vi "ReportExcel20.vi"(1 "Ürün Parça No":string, 2 "Encoder Testi":bool, 3 "Ürün Seri No":string, 4 "Sıcaklık(°C)":dbl, 9 "Test Sonuçlari":string[][](table)=[["Emk Sabiti", "", "1"], ["R1 (U-V)R", "", "2"], ["R2 (V-W)R", "", "3"], ["R3 (U-W)R", "", "4"], ["L1 (U-V)mH", "", "5"], ["L2 (V-W)mH", "", "6"], ["L3 (U-W)mH", "", "7"]] caption="Test Sonuçları", 11 "error in (no error)":errorcluster, 12 "Sonuc":bool, 14 "Faz Doğrulama Testi":bool) -> (10 "appended path":path, 15 "error out":errorcluster)   [LabVIEW 2021]
uses:
  <vilib>/addons/_office/NI_ReportGenerationToolkit.lvlib
  <vilib>/addons/_office/excel.llb/Excel Easy Table (str).vi
  <vilib>/Utility/NIReport.llb/Excel/NI_Excel.lvclass
  <vilib>/Utility/NIReport.llb/NI_report.lvclass
  <vilib>/Utility/NIReport.llb/Report Type.ctl
  <vilib>/Utility/NIReport.llb/NI_ReportGenerationCore.lvlib
  <vilib>/Utility/NIReport.llb/Append Text Table to Report (wrap).vi
  <vilib>/addons/_office/_exclsub.llb/font.ctl
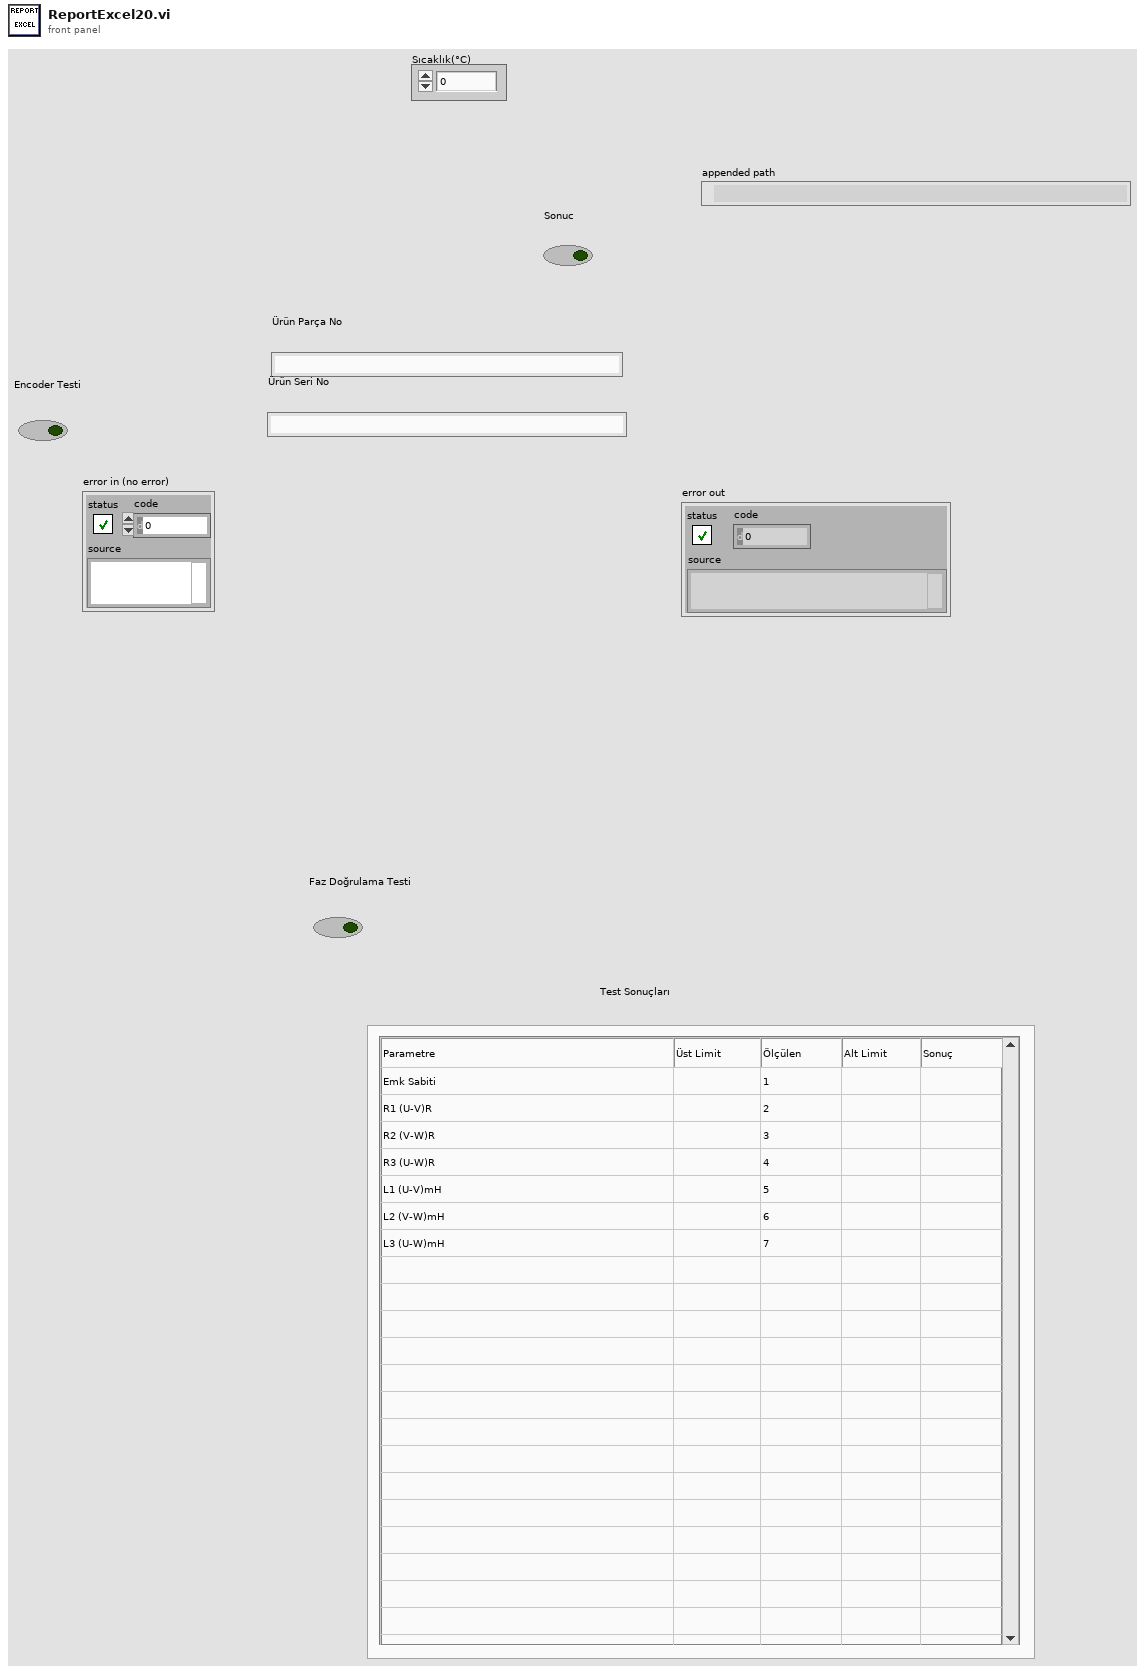
[diagram p1: front panel]
types:
  T1 = typedef "NI_ReportGenerationCore.lvlib/Report Type.ctl" = enum16{"HTML", "Word", "Excel"}
  T2 = enum16{"maximized", "minimized", "normal", "no change"}
  T3 = typedef "NI_ReportGenerationToolkit.lvlib/font.ctl" = cluster{"font name":string, "font size":dbl, "bold":u16, "italic":u16, "underline":u16, "strike through":u16, "font color":u32}
  T4 = cluster{"position (excel)":cluster{"row":i32, "column":i32}, "name (excel)":string, "bookmark (word)":string}
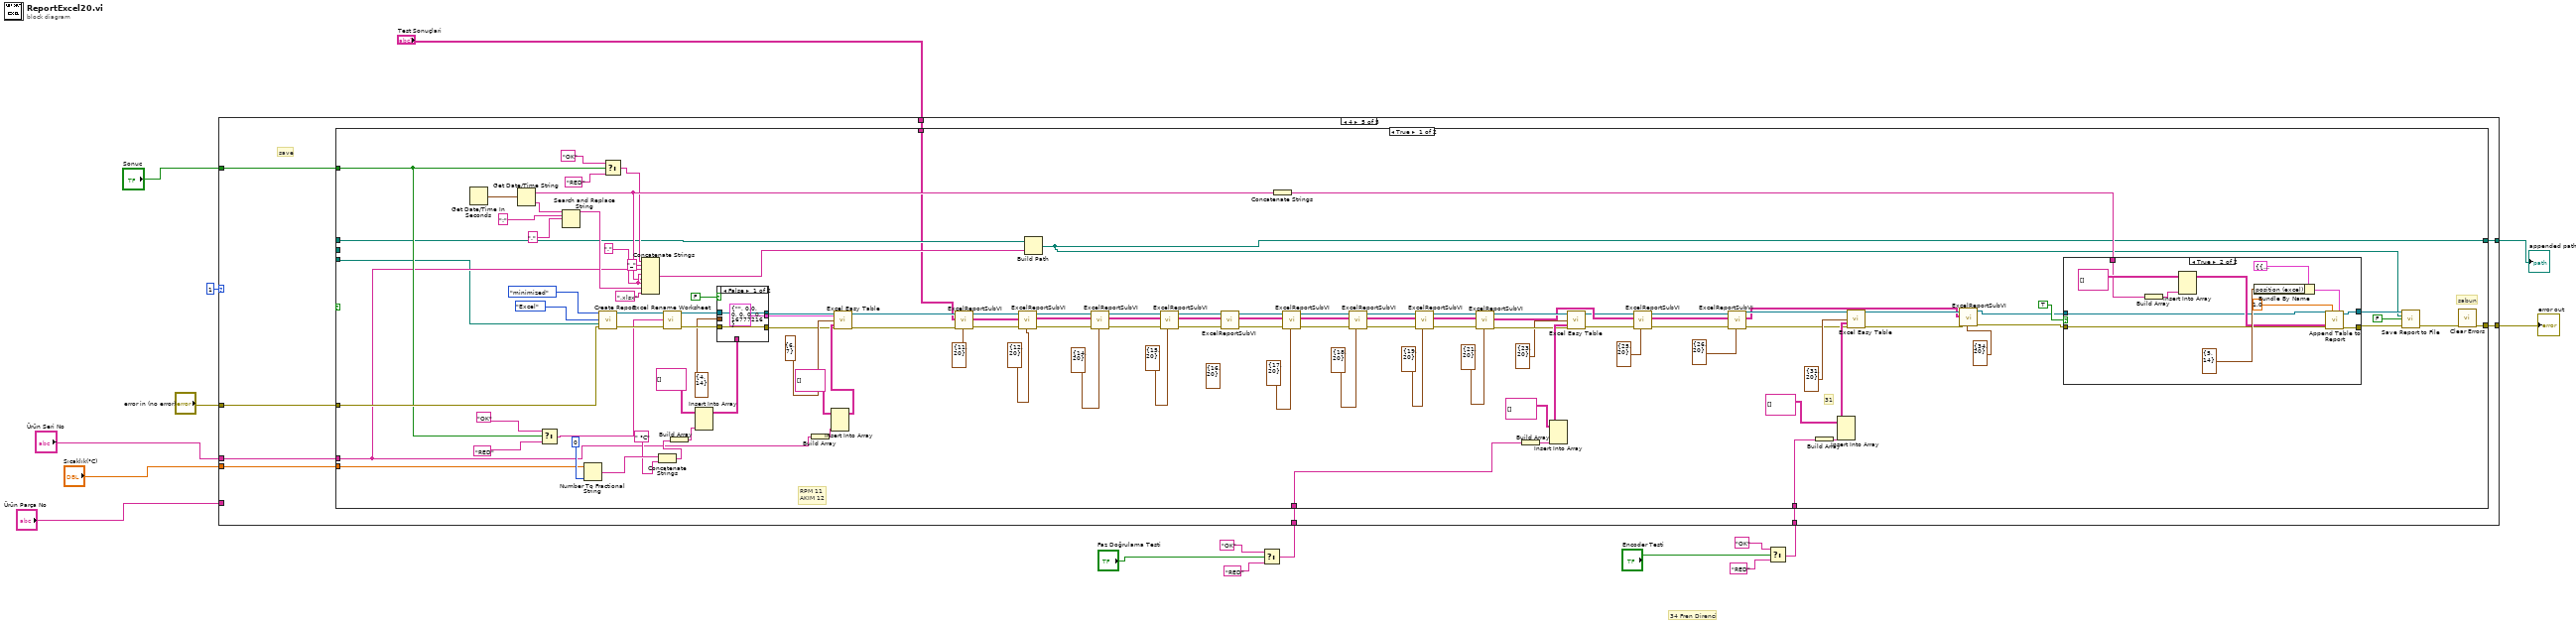
[diagram p0: block diagram]
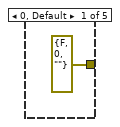
[diagram p2: hidden frame]
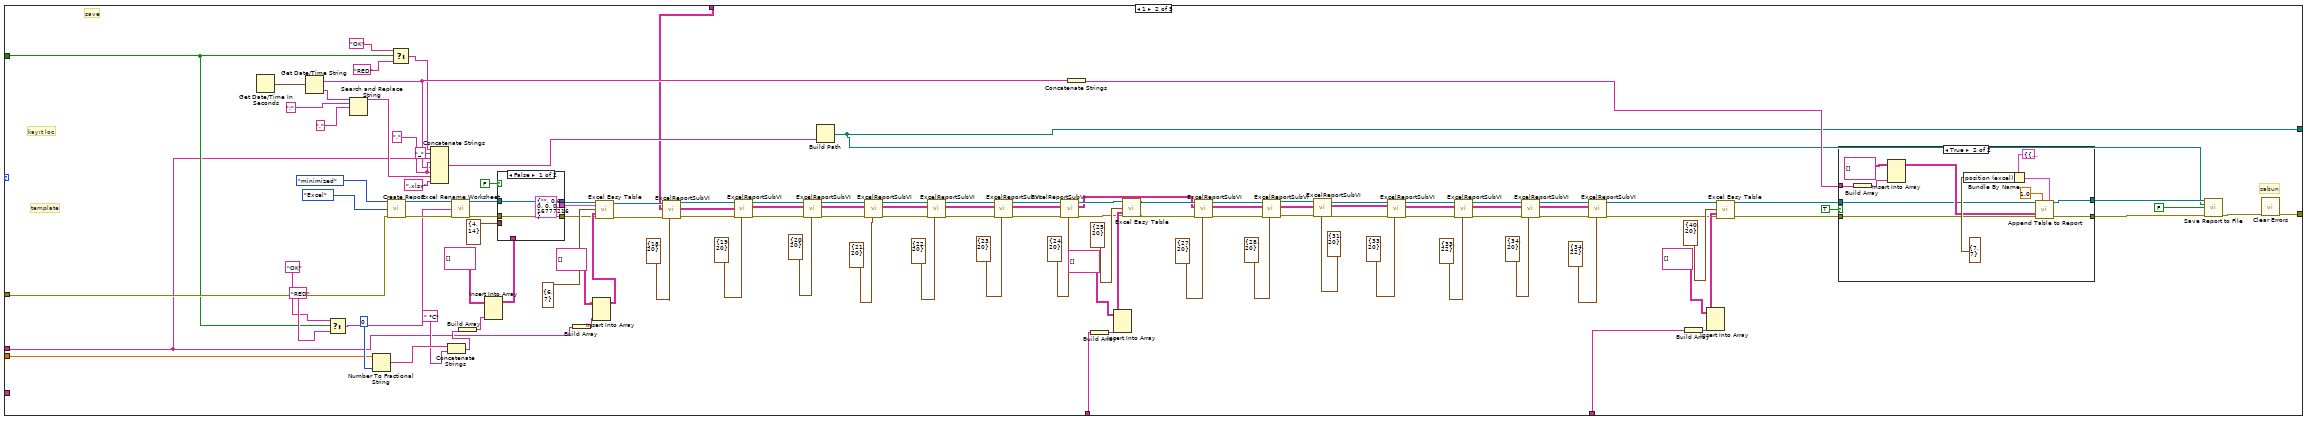
[diagram p3: hidden frame]
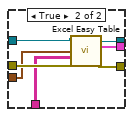
[diagram p4: hidden frame]
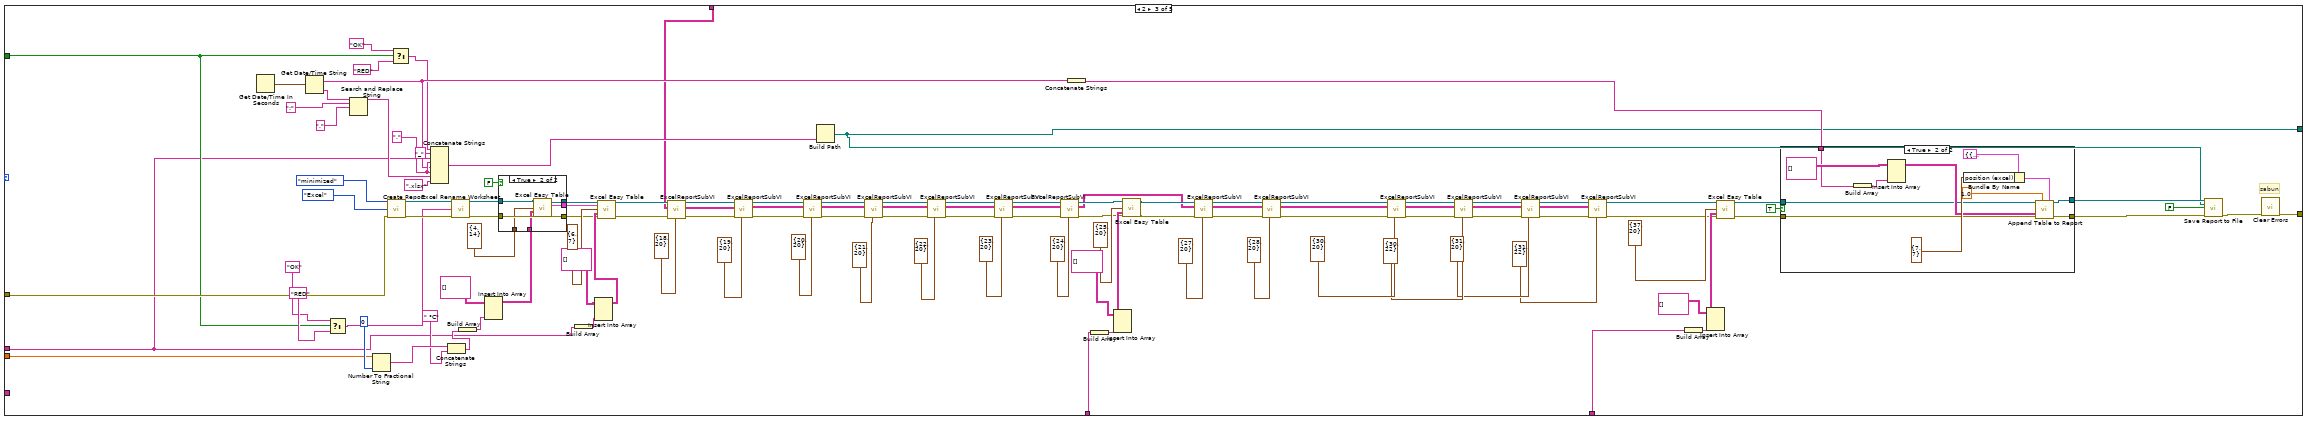
[diagram p6: hidden frame]
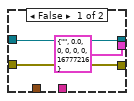
[diagram p7: hidden frame]
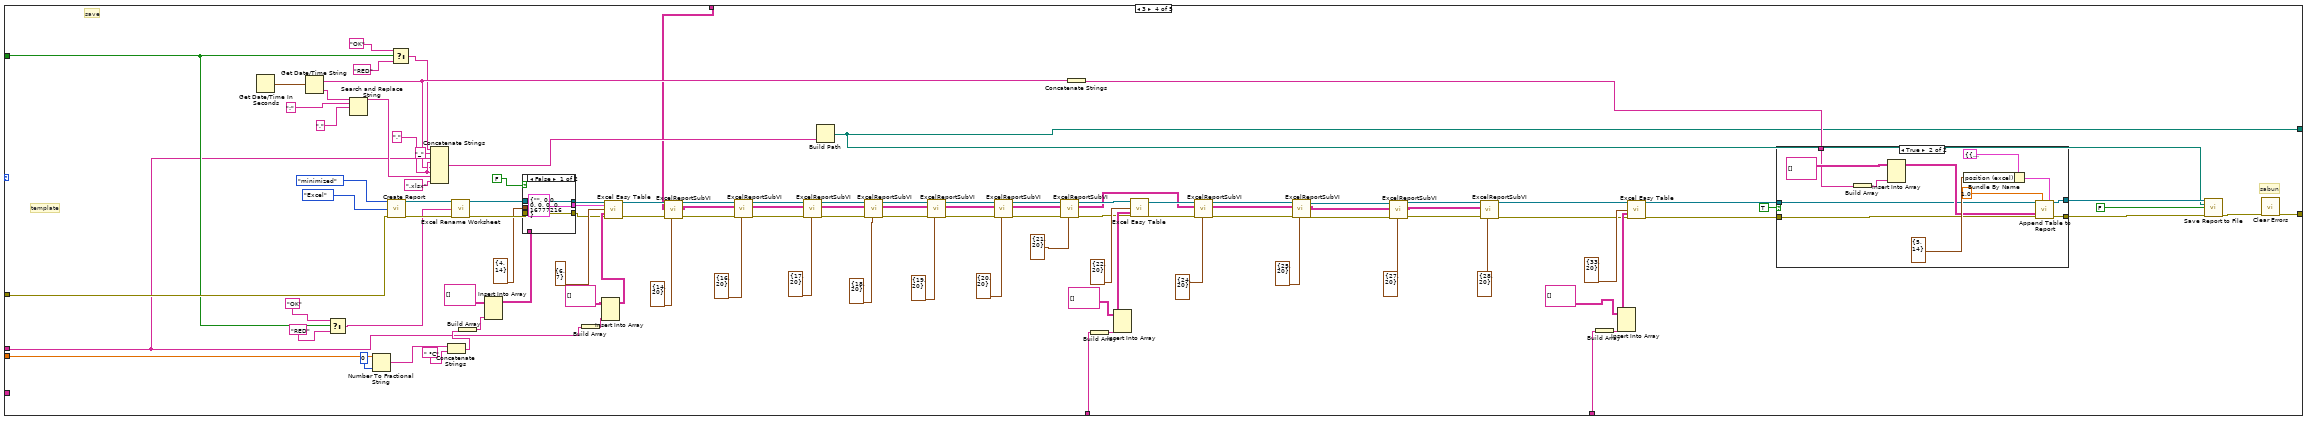
[diagram p9: hidden frame]
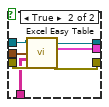
[diagram p10: hidden frame]
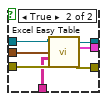
[diagram p12: hidden frame]
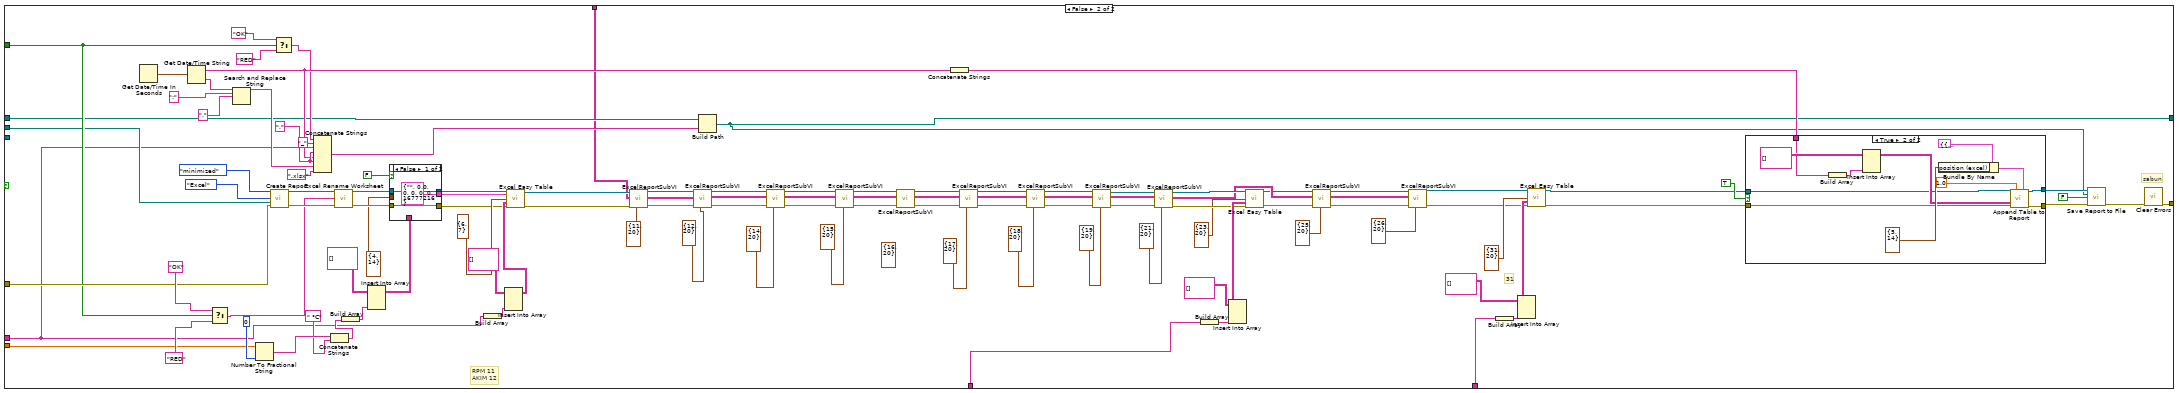
[diagram p14: hidden frame]
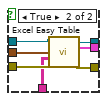
[diagram p15: hidden frame]
diagram:
  # "34 Fren Direnci"
  n1 = Select(t="OK" ("worksheet name (\"\")"), s="Faz Doğrulama Testi", f="RED" ("worksheet name (\"\")")) -> (s? t:f=w13:string)
  n2 = Select(t="OK" ("worksheet name (\"\")"), s="Encoder Testi", f="RED" ("worksheet name (\"\")")) -> (s? t:f=w12:string)
  n3 = case shown="4" 1 {
    tunnel: [errorcluster {"status"=FALSE, "code"=0, "source"=""} ("error out") w108 w252 w398 w466] -> w17
    tunnel: w13 -> [_ w74 w216 w371 w459]
    tunnel: w12 -> [_ w66 w208 w363 w458]
    tunnel: "Sıcaklık(°C)" -> [_ w54 w196 w346 w465]
    tunnel: "error in (no error)" -> [_ w53 w195 w345 w464]
    tunnel: "Sonuc" -> [_ w52 w194 w344 w463]
    tunnel: [_ w51 w193 w343 w462] -> w5
    tunnel: "Ürün Seri No" -> [_ w40 w187 w327 w460]
    tunnel: "Ürün Parça No" -> [_ _ _ _ _]
    tunnel: "Test Sonuçlari" -> [_ w34 w179 w324 w461]
    frame 0, Default {
    }
    frame 1 {
      w132 = "." ("string")
      # "kayıt loc"
      # "save"
      # "template"
      # "sabun"
      n4 = Get Date/Time In Seconds() -> (seconds since 1Jan1904=w139:timestamp)
      n5 = Get Date/Time String(seconds (now)=w139) -> (date string=w129:string, time string=w130:string)  [unwired: 2 in]
      n6 = Select(t="OK" ("worksheet name (\"\")"), s=w52, f="RED" ("worksheet name (\"\")")) -> (s? t:f=w131:string)
      n7 = Search and Replace String(input string=w130, search string=":", replace string="." ("replace string (\"\")")) -> (result string=w125:string)  [unwired: 5 in, 3 out]
      n8 = Number To Fractional String(number=w54, precision (6)=i16 0) -> (F-format string=w115:string)  [unwired: 2 in]
      n9 = call <vilib>:"Create Report.vi"("window state (normal)"=T2."minimized", "report type"=Report_Type."Excel", "error in (no error)"=w53) -> ("report out"=w141:refnum<class "NI_report.lvclass">, "template (empty)"=w49:path, "error out"=w140:errorcluster)  [unwired: 10 in]
      n10 = Select(t="OK" ("worksheet name (\"\")"), s=w52, f="RED" ("worksheet name (\"\")")) -> (s? t:f=w55:string)
      n11 = Concatenate Strings(w55, "_" ("string"), w40, w132, w129, w132, w125, ".xlsx" ("string")) -> (w136:string)
      n12 = Concatenate Strings(w115, " °C" ("string")) -> (w113:string)
      n13 = call <vilib>:"Excel Rename Worksheet.vi"("report in"=w141, "worksheet name (\"\")"=w131, "error in (no error)"=w140) -> ("report out"=w120:refnum<class "NI_report.lvclass">, "error out"=w119:errorcluster)  [unwired: 11 in]
      n14 = Build Array(w113) -> (w116:string[])
      n15 = Insert Into Array(array=string[][] [] ("text data"), new element=w116) -> (w112:string[][])  [unwired: 2 in]
      n16 = case shown="False" FALSE {
        tunnel: w120 -> [w145 w152]
        tunnel: w119 -> [w144 w151]
        tunnel: cluster{"row":i32, "column":i32} {"row"=4, "column"=14} ("start (0, 0)") -> [_ w150]
        tunnel: w112 -> [_ w149]
        tunnel: [w145 w148] -> w43
        tunnel: [w144 w147] -> w42
        tunnel: [T3 {"font name"="", "font size"=0.0, "bold"=0, "italic"=0, "underline"=0, "strike through"=0, "font color"=16777216} ("font out") w146] -> w41
        frame False {
        }
        frame True {
          n17 = call-poly <vilib>:"Excel Easy Table.vi"("report in"=w152, "start (0, 0)"=w150, "text data"=w149, "error in (no error)"=w151) -> ("report out"=w148:refnum<class "NI_report.lvclass">, "font out"=w146:T3, "error out"=w147:errorcluster)  [unwired: 7 in, 2 out]
        }
      }
      n18 = Build Array(w40) -> (w124:string[])
      n19 = Insert Into Array(array=string[][] [] ("text data"), new element=w124) -> (w123:string[][])  [unwired: 2 in]
      n20 = call-poly <vilib>:"Excel Easy Table.vi"("report in"=w43, "font"=w41, "start (0, 0)"=cluster{"row":i32, "column":i32} {"row"=6, "column"=7}, "text data"=w123, "error in (no error)"=w42) -> ("report out"=w38:refnum<class "NI_report.lvclass">, "error out"=w37:errorcluster)  [unwired: 6 in, 3 out]
      n21 = call "ExcelReportSubVI.vi"("start (0, 0)"=cluster{"row":i32, "column":i32} {"row"=18, "column"=20}, "error in (no error)"=w37, "Test İn"=w34, "report in"=w38) -> ("error out"=w35:errorcluster, "Table out"=w33:string[][], "report out"=w36:refnum<class "NI_report.lvclass">)  [unwired: 5 in]
      n22 = call "ExcelReportSubVI.vi"("start (0, 0)"=cluster{"row":i32, "column":i32} {"row"=19, "column"=20}, "error in (no error)"=w35, "Test İn"=w33, "report in"=w36) -> ("error out"=w106:errorcluster, "Table out"=w32:string[][], "report out"=w107:refnum<class "NI_report.lvclass">)  [unwired: 5 in]
      n23 = call "ExcelReportSubVI.vi"("start (0, 0)"=cluster{"row":i32, "column":i32} {"row"=20, "column"=20}, "error in (no error)"=w106, "Test İn"=w32, "report in"=w107) -> ("error out"=w104:errorcluster, "Table out"=w31:string[][], "report out"=w105:refnum<class "NI_report.lvclass">)  [unwired: 5 in]
      n24 = Build Path(name or relative path=w136) -> (base path=w50:path, appended path=w51:path)
      n25 = call "ExcelReportSubVI.vi"("start (0, 0)"=cluster{"row":i32, "column":i32} {"row"=21, "column"=20}, "error in (no error)"=w104, "Test İn"=w31, "report in"=w105) -> ("error out"=w96:errorcluster, "Table out"=w30:string[][], "report out"=w103:refnum<class "NI_report.lvclass">)  [unwired: 5 in]
      n26 = call "ExcelReportSubVI.vi"("start (0, 0)"=cluster{"row":i32, "column":i32} {"row"=22, "column"=20}, "error in (no error)"=w96, "Test İn"=w30, "report in"=w103) -> ("error out"=w95:errorcluster, "Table out"=w29:string[][], "report out"=w102:refnum<class "NI_report.lvclass">)  [unwired: 5 in]
      n27 = call "ExcelReportSubVI.vi"("start (0, 0)"=cluster{"row":i32, "column":i32} {"row"=23, "column"=20}, "error in (no error)"=w95, "Test İn"=w29, "report in"=w102) -> ("error out"=w94:errorcluster, "Table out"=w28:string[][], "report out"=w101:refnum<class "NI_report.lvclass">)  [unwired: 5 in]
      n28 = call "ExcelReportSubVI.vi"("start (0, 0)"=cluster{"row":i32, "column":i32} {"row"=24, "column"=20}, "error in (no error)"=w94, "Test İn"=w28, "report in"=w101) -> ("error out"=w71:errorcluster, "Table out"=w27:string[][], "report out"=w72:refnum<class "NI_report.lvclass">)  [unwired: 5 in]
      n29 = Concatenate Strings(w129) -> (w128:string)
      n30 = Build Array(w74) -> (w75:string[])
      n31 = Insert Into Array(array=string[][] [] ("text data"), new element=w75) -> (w77:string[][])  [unwired: 2 in]
      n32 = call-poly <vilib>:"Excel Easy Table.vi"("report in"=w72, "start (0, 0)"=cluster{"row":i32, "column":i32} {"row"=25, "column"=20}, "text data"=w77, "error in (no error)"=w71) -> ("report out"=w69:refnum<class "NI_report.lvclass">, "error out"=w70:errorcluster)  [unwired: 7 in, 3 out]
      n33 = call "ExcelReportSubVI.vi"("start (0, 0)"=cluster{"row":i32, "column":i32} {"row"=27, "column"=20}, "error in (no error)"=w70, "Test İn"=w27, "report in"=w69) -> ("error out"=w93:errorcluster, "Table out"=w26:string[][], "report out"=w100:refnum<class "NI_report.lvclass">)  [unwired: 5 in]
      n34 = call "ExcelReportSubVI.vi"("start (0, 0)"=cluster{"row":i32, "column":i32} {"row"=28, "column"=20}, "error in (no error)"=w93, "Test İn"=w26, "report in"=w100) -> ("error out"=w47:errorcluster, "Table out"=w25:string[][], "report out"=w48:refnum<class "NI_report.lvclass">)  [unwired: 5 in]
      n35 = call "ExcelReportSubVI.vi"("start (0, 0)"=cluster{"row":i32, "column":i32} {"row"=31, "column"=20}, "error in (no error)"=w47, "Test İn"=w25, "report in"=w48) -> ("error out"=w45:errorcluster, "Table out"=w24:string[][], "report out"=w46:refnum<class "NI_report.lvclass">)  [unwired: 5 in]
      n36 = call "ExcelReportSubVI.vi"("start (0, 0)"=cluster{"row":i32, "column":i32} {"row"=33, "column"=20}, "error in (no error)"=w45, "Test İn"=w24, "report in"=w46) -> ("error out"=w92:errorcluster, "Table out"=w23:string[][], "report out"=w99:refnum<class "NI_report.lvclass">)  [unwired: 5 in]
      n37 = call "ExcelReportSubVI.vi"("start (0, 0)"=cluster{"row":i32, "column":i32} {"row"=33, "column"=22}, "error in (no error)"=w92, "Test İn"=w23, "report in"=w99) -> ("error out"=w91:errorcluster, "Table out"=w22:string[][], "report out"=w98:refnum<class "NI_report.lvclass">)  [unwired: 5 in]
      n38 = call "ExcelReportSubVI.vi"("start (0, 0)"=cluster{"row":i32, "column":i32} {"row"=34, "column"=20}, "error in (no error)"=w91, "Test İn"=w22, "report in"=w98) -> ("error out"=w90:errorcluster, "Table out"=w21:string[][], "report out"=w97:refnum<class "NI_report.lvclass">)  [unwired: 5 in]
      n39 = call "ExcelReportSubVI.vi"("start (0, 0)"=cluster{"row":i32, "column":i32} {"row"=34, "column"=22}, "error in (no error)"=w90, "Test İn"=w21, "report in"=w97) -> ("error out"=w61:errorcluster, "report out"=w62:refnum<class "NI_report.lvclass">)  [unwired: 5 in, 1 out]
      n40 = Build Array(w66) -> (w65:string[])
      n41 = Insert Into Array(array=string[][] [] ("text data"), new element=w65) -> (w63:string[][])  [unwired: 2 in]
      n42 = call-poly <vilib>:"Excel Easy Table.vi"("report in"=w62, "start (0, 0)"=cluster{"row":i32, "column":i32} {"row"=40, "column"=20}, "text data"=w63, "error in (no error)"=w61) -> ("report out"=w60:refnum<class "NI_report.lvclass">, "error out"=w59:errorcluster)  [unwired: 7 in, 3 out]
      n43 = case shown="True" TRUE {
        tunnel: w128 -> [_ w164]
        tunnel: [w154 w158] -> w127
        tunnel: [w153 w157] -> w126
        tunnel: w60 -> [w154 w156]
        tunnel: w59 -> [w153 w155]
        frame False {
        }
        frame True {
          n44 = Build Array(w164) -> (w165:string[])
          n45 = Insert Into Array(array=string[][] [] ("text data"), new element=w165) -> (w159:string[][])  [unwired: 2 in]
          n46 = Bundle By Name(cluster=T4 {"position (excel)"={"row"=0, "column"=0}, "name (excel)"="", "bookmark (word)"=""} ("MS Office parameters"), "position (excel)"=cluster{"row":i32, "column":i32} {"row"=7, "column"=7} ("start (0, 0)")) -> (w161:T4)
          n47 = call-poly <vilib>:"Append Table to Report.vi"("report in"=w156, "column width (1)"=1.0, "MS Office parameters"=w161, "text data"=w159, "error in (no error)"=w155) -> ("report out"=w158:refnum<class "NI_report.lvclass">, "error out"=w157:errorcluster)  [unwired: 7 in, 2 out]
        }
      }
      n48 = call-dynamic "Save Report to File.vi"("report in"=w127, "report file path"=w51, "prompt to replace? (F)"=FALSE, "error in (no error)"=w126) -> ("error out"=w109:errorcluster)  [unwired: 10 in, 1 out]
      n49 = call <vilib>:"Clear Errors.vi"("error in (no error)"=w109) -> ("error out"=w108:errorcluster)  [unwired: 5 in, 1 out]
    }
    frame 2 {
      w276 = "." ("string")
      # "sabun"
      n50 = Get Date/Time In Seconds() -> (seconds since 1Jan1904=w283:timestamp)
      n51 = Get Date/Time String(seconds (now)=w283) -> (date string=w273:string, time string=w274:string)  [unwired: 2 in]
      n52 = Select(t="OK" ("worksheet name (\"\")"), s=w194, f="RED" ("worksheet name (\"\")")) -> (s? t:f=w275:string)
      n53 = Search and Replace String(input string=w274, search string=":", replace string="." ("replace string (\"\")")) -> (result string=w269:string)  [unwired: 5 in, 3 out]
      n54 = Number To Fractional String(number=w196, precision (6)=i16 0) -> (F-format string=w259:string)  [unwired: 2 in]
      n55 = call <vilib>:"Create Report.vi"("window state (normal)"=T2."minimized", "report type"=Report_Type."Excel", "error in (no error)"=w195) -> ("report out"=w285:refnum<class "NI_report.lvclass">, "template (empty)"=w191:path, "error out"=w284:errorcluster)  [unwired: 10 in]
      n56 = Select(t="OK" ("worksheet name (\"\")"), s=w194, f="RED" ("worksheet name (\"\")")) -> (s? t:f=w197:string)
      n57 = Concatenate Strings(w197, "_" ("string"), w187, w276, w273, w276, w269, ".xlsx" ("string")) -> (w280:string)
      n58 = Concatenate Strings(w259, " °C" ("string")) -> (w257:string)
      n59 = call <vilib>:"Excel Rename Worksheet.vi"("report in"=w285, "worksheet name (\"\")"=w275, "error in (no error)"=w284) -> ("report out"=w264:refnum<class "NI_report.lvclass">, "error out"=w263:errorcluster)  [unwired: 11 in]
      n60 = Build Array(w257) -> (w260:string[])
      n61 = Insert Into Array(array=string[][] [] ("text data"), new element=w260) -> (w256:string[][])  [unwired: 2 in]
      n62 = case shown="True" FALSE {
        tunnel: w264 -> [w289 w296]
        tunnel: w263 -> [w288 w295]
        tunnel: cluster{"row":i32, "column":i32} {"row"=4, "column"=14} ("start (0, 0)") -> [_ w294]
        tunnel: w256 -> [_ w293]
        tunnel: [w289 w292] -> w190
        tunnel: [w288 w291] -> w189
        tunnel: [T3 {"font name"="", "font size"=0.0, "bold"=0, "italic"=0, "underline"=0, "strike through"=0, "font color"=16777216} ("font out") w290] -> w188
        frame False {
        }
        frame True {
          n63 = call-poly <vilib>:"Excel Easy Table.vi"("report in"=w296, "start (0, 0)"=w294, "text data"=w293, "error in (no error)"=w295) -> ("report out"=w292:refnum<class "NI_report.lvclass">, "font out"=w290:T3, "error out"=w291:errorcluster)  [unwired: 7 in, 2 out]
        }
      }
      n64 = Build Array(w187) -> (w268:string[])
      n65 = Insert Into Array(array=string[][] [] ("text data"), new element=w268) -> (w267:string[][])  [unwired: 2 in]
      n66 = call-poly <vilib>:"Excel Easy Table.vi"("report in"=w190, "font"=w188, "start (0, 0)"=cluster{"row":i32, "column":i32} {"row"=6, "column"=7}, "text data"=w267, "error in (no error)"=w189) -> ("report out"=w185:refnum<class "NI_report.lvclass">, "error out"=w183:errorcluster)  [unwired: 6 in, 3 out]
      n67 = call "ExcelReportSubVI.vi"("start (0, 0)"=cluster{"row":i32, "column":i32} {"row"=18, "column"=20}, "error in (no error)"=w183, "Test İn"=w179, "report in"=w185) -> ("error out"=w182:errorcluster, "Table out"=w180:string[][], "report out"=w184:refnum<class "NI_report.lvclass">)  [unwired: 5 in]
      n68 = call "ExcelReportSubVI.vi"("start (0, 0)"=cluster{"row":i32, "column":i32} {"row"=19, "column"=20}, "error in (no error)"=w182, "Test İn"=w180, "report in"=w184) -> ("error out"=w250:errorcluster, "Table out"=w178:string[][], "report out"=w251:refnum<class "NI_report.lvclass">)  [unwired: 5 in]
      n69 = call "ExcelReportSubVI.vi"("start (0, 0)"=cluster{"row":i32, "column":i32} {"row"=20, "column"=20}, "error in (no error)"=w250, "Test İn"=w178, "report in"=w251) -> ("error out"=w248:errorcluster, "Table out"=w177:string[][], "report out"=w249:refnum<class "NI_report.lvclass">)  [unwired: 5 in]
      n70 = Build Path(name or relative path=w280) -> (base path=w192:path, appended path=w193:path)
      n71 = call "ExcelReportSubVI.vi"("start (0, 0)"=cluster{"row":i32, "column":i32} {"row"=21, "column"=20}, "error in (no error)"=w248, "Test İn"=w177, "report in"=w249) -> ("error out"=w239:errorcluster, "Table out"=w176:string[][], "report out"=w247:refnum<class "NI_report.lvclass">)  [unwired: 5 in]
      n72 = call "ExcelReportSubVI.vi"("start (0, 0)"=cluster{"row":i32, "column":i32} {"row"=22, "column"=20}, "error in (no error)"=w239, "Test İn"=w176, "report in"=w247) -> ("error out"=w238:errorcluster, "Table out"=w175:string[][], "report out"=w246:refnum<class "NI_report.lvclass">)  [unwired: 5 in]
      n73 = call "ExcelReportSubVI.vi"("start (0, 0)"=cluster{"row":i32, "column":i32} {"row"=23, "column"=20}, "error in (no error)"=w238, "Test İn"=w175, "report in"=w246) -> ("error out"=w237:errorcluster, "Table out"=w174:string[][], "report out"=w245:refnum<class "NI_report.lvclass">)  [unwired: 5 in]
      n74 = call "ExcelReportSubVI.vi"("start (0, 0)"=cluster{"row":i32, "column":i32} {"row"=24, "column"=20}, "error in (no error)"=w237, "Test İn"=w174, "report in"=w245) -> ("error out"=w213:errorcluster, "Table out"=w173:string[][], "report out"=w214:refnum<class "NI_report.lvclass">)  [unwired: 5 in]
      n75 = Concatenate Strings(w273) -> (w272:string)
      n76 = Build Array(w216) -> (w217:string[])
      n77 = Insert Into Array(array=string[][] [] ("text data"), new element=w217) -> (w219:string[][])  [unwired: 2 in]
      n78 = call-poly <vilib>:"Excel Easy Table.vi"("report in"=w214, "start (0, 0)"=cluster{"row":i32, "column":i32} {"row"=25, "column"=20}, "text data"=w219, "error in (no error)"=w213) -> ("report out"=w211:refnum<class "NI_report.lvclass">, "error out"=w212:errorcluster)  [unwired: 7 in, 3 out]
      n79 = call "ExcelReportSubVI.vi"("start (0, 0)"=cluster{"row":i32, "column":i32} {"row"=27, "column"=20}, "error in (no error)"=w212, "Test İn"=w173, "report in"=w211) -> ("error out"=w236:errorcluster, "Table out"=w172:string[][], "report out"=w244:refnum<class "NI_report.lvclass">)  [unwired: 5 in]
      n80 = call "ExcelReportSubVI.vi"("start (0, 0)"=cluster{"row":i32, "column":i32} {"row"=28, "column"=20}, "error in (no error)"=w236, "Test İn"=w172, "report in"=w244) -> ("error out"=w235:errorcluster, "Table out"=w171:string[][], "report out"=w243:refnum<class "NI_report.lvclass">)  [unwired: 5 in]
      n81 = call "ExcelReportSubVI.vi"("start (0, 0)"=cluster{"row":i32, "column":i32} {"row"=30, "column"=20}, "error in (no error)"=w235, "Test İn"=w171, "report in"=w243) -> ("error out"=w234:errorcluster, "Table out"=w170:string[][], "report out"=w242:refnum<class "NI_report.lvclass">)  [unwired: 5 in]
      n82 = call "ExcelReportSubVI.vi"("start (0, 0)"=cluster{"row":i32, "column":i32} {"row"=30, "column"=22}, "error in (no error)"=w234, "Test İn"=w170, "report in"=w242) -> ("error out"=w233:errorcluster, "Table out"=w169:string[][], "report out"=w241:refnum<class "NI_report.lvclass">)  [unwired: 5 in]
      n83 = call "ExcelReportSubVI.vi"("start (0, 0)"=cluster{"row":i32, "column":i32} {"row"=31, "column"=20}, "error in (no error)"=w233, "Test İn"=w169, "report in"=w241) -> ("error out"=w232:errorcluster, "Table out"=w168:string[][], "report out"=w240:refnum<class "NI_report.lvclass">)  [unwired: 5 in]
      n84 = call "ExcelReportSubVI.vi"("start (0, 0)"=cluster{"row":i32, "column":i32} {"row"=31, "column"=22}, "error in (no error)"=w232, "Test İn"=w168, "report in"=w240) -> ("error out"=w203:errorcluster, "report out"=w204:refnum<class "NI_report.lvclass">)  [unwired: 5 in, 1 out]
      n85 = Build Array(w208) -> (w207:string[])
      n86 = Insert Into Array(array=string[][] [] ("text data"), new element=w207) -> (w205:string[][])  [unwired: 2 in]
      n87 = call-poly <vilib>:"Excel Easy Table.vi"("report in"=w204, "start (0, 0)"=cluster{"row":i32, "column":i32} {"row"=37, "column"=20}, "text data"=w205, "error in (no error)"=w203) -> ("report out"=w202:refnum<class "NI_report.lvclass">, "error out"=w201:errorcluster)  [unwired: 7 in, 3 out]
      n88 = case shown="True" TRUE {
        tunnel: w272 -> [_ w308]
        tunnel: [w298 w302] -> w271
        tunnel: [w297 w301] -> w270
        tunnel: w202 -> [w298 w300]
        tunnel: w201 -> [w297 w299]
        frame False {
        }
        frame True {
          n89 = Build Array(w308) -> (w309:string[])
          n90 = Insert Into Array(array=string[][] [] ("text data"), new element=w309) -> (w303:string[][])  [unwired: 2 in]
          n91 = Bundle By Name(cluster=T4 {"position (excel)"={"row"=0, "column"=0}, "name (excel)"="", "bookmark (word)"=""} ("MS Office parameters"), "position (excel)"=cluster{"row":i32, "column":i32} {"row"=7, "column"=7} ("start (0, 0)")) -> (w305:T4)
          n92 = call-poly <vilib>:"Append Table to Report.vi"("report in"=w300, "column width (1)"=1.0, "MS Office parameters"=w305, "text data"=w303, "error in (no error)"=w299) -> ("report out"=w302:refnum<class "NI_report.lvclass">, "error out"=w301:errorcluster)  [unwired: 7 in, 2 out]
        }
      }
      n93 = call-dynamic "Save Report to File.vi"("report in"=w271, "report file path"=w193, "prompt to replace? (F)"=FALSE, "error in (no error)"=w270) -> ("error out"=w253:errorcluster)  [unwired: 10 in, 1 out]
      n94 = call <vilib>:"Clear Errors.vi"("error in (no error)"=w253) -> ("error out"=w252:errorcluster)  [unwired: 5 in, 1 out]
    }
    frame 3 {
      w421 = "." ("string")
      # "save"
      # "template"
      # "sabun"
      n95 = Get Date/Time In Seconds() -> (seconds since 1Jan1904=w428:timestamp)
      n96 = Get Date/Time String(seconds (now)=w428) -> (date string=w419:string, time string=w311:string)  [unwired: 2 in]
      n97 = Select(t="OK" ("worksheet name (\"\")"), s=w344, f="RED" ("worksheet name (\"\")")) -> (s? t:f=w420:string)
      n98 = Search and Replace String(input string=w311, search string=":", replace string="." ("replace string (\"\")")) -> (result string=w415:string)  [unwired: 5 in, 3 out]
      n99 = Number To Fractional String(number=w346, precision (6)=i16 0) -> (F-format string=w405:string)  [unwired: 2 in]
      n100 = call <vilib>:"Create Report.vi"("window state (normal)"=T2."minimized", "report type"=Report_Type."Excel", "error in (no error)"=w345) -> ("report out"=w430:refnum<class "NI_report.lvclass">, "template (empty)"=w341:path, "error out"=w429:errorcluster)  [unwired: 10 in]
      n101 = Select(t="OK" ("worksheet name (\"\")"), s=w344, f="RED" ("worksheet name (\"\")")) -> (s? t:f=w354:string)
      n102 = Concatenate Strings(w354, "_" ("string"), w327, w421, w419, w421, w415, ".xlsx" ("string")) -> (w425:string)
      n103 = Concatenate Strings(w405, " °C" ("string")) -> (w403:string)
      n104 = call <vilib>:"Excel Rename Worksheet.vi"("report in"=w430, "worksheet name (\"\")"=w420, "error in (no error)"=w429) -> ("report out"=w410:refnum<class "NI_report.lvclass">, "error out"=w409:errorcluster)  [unwired: 11 in]
      n105 = Build Array(w403) -> (w406:string[])
      n106 = Insert Into Array(array=string[][] [] ("text data"), new element=w406) -> (w402:string[][])  [unwired: 2 in]
      n107 = case shown="False" FALSE {
        tunnel: w410 -> [w434 w441]
        tunnel: w409 -> [w433 w440]
        tunnel: cluster{"row":i32, "column":i32} {"row"=4, "column"=14} ("start (0, 0)") -> [_ w439]
        tunnel: w402 -> [_ w438]
        tunnel: [w434 w437] -> w330
        tunnel: [w433 w436] -> w329
        tunnel: [T3 {"font name"="", "font size"=0.0, "bold"=0, "italic"=0, "underline"=0, "strike through"=0, "font color"=16777216} ("font out") w435] -> w328
        frame False {
        }
        frame True {
          n108 = call-poly <vilib>:"Excel Easy Table.vi"("report in"=w441, "start (0, 0)"=w439, "text data"=w438, "error in (no error)"=w440) -> ("report out"=w437:refnum<class "NI_report.lvclass">, "font out"=w435:T3, "error out"=w436:errorcluster)  [unwired: 7 in, 2 out]
        }
      }
      n109 = Build Array(w327) -> (w414:string[])
      n110 = Insert Into Array(array=string[][] [] ("text data"), new element=w414) -> (w413:string[][])  [unwired: 2 in]
      n111 = call-poly <vilib>:"Excel Easy Table.vi"("report in"=w330, "font"=w328, "start (0, 0)"=cluster{"row":i32, "column":i32} {"row"=6, "column"=7}, "text data"=w413, "error in (no error)"=w329) -> ("report out"=w397:refnum<class "NI_report.lvclass">, "error out"=w396:errorcluster)  [unwired: 6 in, 3 out]
      n112 = call "ExcelReportSubVI.vi"("start (0, 0)"=cluster{"row":i32, "column":i32} {"row"=14, "column"=20}, "Test İn"=w324) -> ("Table out"=w323:string[][], "Yazılacak Parametre"=w325:string)  [unwired: 6 in, 2 out]
      n113 = call "ExcelReportSubVI.vi"("start (0, 0)"=cluster{"row":i32, "column":i32} {"row"=16, "column"=20}, "error in (no error)"=w396, "Test İn"=w323, "report in"=w397) -> ("error out"=w394:errorcluster, "Table out"=w322:string[][], "report out"=w395:refnum<class "NI_report.lvclass">, "Yazılacak Parametre"=w353:string)  [unwired: 4 in]
      n114 = call "ExcelReportSubVI.vi"("start (0, 0)"=cluster{"row":i32, "column":i32} {"row"=17, "column"=20}, "error in (no error)"=w394, "Test İn"=w322, "report in"=w395) -> ("error out"=w392:errorcluster, "Table out"=w321:string[][], "report out"=w393:refnum<class "NI_report.lvclass">, "Yazılacak Parametre"=w352:string)  [unwired: 4 in]
      n115 = Build Path(name or relative path=w425) -> (base path=w342:path, appended path=w343:path)
      n116 = call "ExcelReportSubVI.vi"("start (0, 0)"=cluster{"row":i32, "column":i32} {"row"=18, "column"=20}, "error in (no error)"=w392, "Test İn"=w321, "report in"=w393) -> ("error out"=w387:errorcluster, "Table out"=w320:string[][], "report out"=w391:refnum<class "NI_report.lvclass">, "Yazılacak Parametre"=w351:string)  [unwired: 4 in]
      n117 = call "ExcelReportSubVI.vi"("start (0, 0)"=cluster{"row":i32, "column":i32} {"row"=19, "column"=20}, "error in (no error)"=w387, "Test İn"=w320, "report in"=w391) -> ("error out"=w386:errorcluster, "Table out"=w319:string[][], "report out"=w390:refnum<class "NI_report.lvclass">, "Yazılacak Parametre"=w350:string)  [unwired: 4 in]
      n118 = call "ExcelReportSubVI.vi"("start (0, 0)"=cluster{"row":i32, "column":i32} {"row"=20, "column"=20}, "error in (no error)"=w386, "Test İn"=w319, "report in"=w390) -> ("error out"=w385:errorcluster, "Table out"=w318:string[][], "report out"=w389:refnum<class "NI_report.lvclass">, "Yazılacak Parametre"=w349:string)  [unwired: 4 in]
      n119 = call "ExcelReportSubVI.vi"("start (0, 0)"=cluster{"row":i32, "column":i32} {"row"=21, "column"=20}, "error in (no error)"=w385, "Test İn"=w318, "report in"=w389) -> ("error out"=w368:errorcluster, "Table out"=w317:string[][], "report out"=w369:refnum<class "NI_report.lvclass">, "Yazılacak Parametre"=w348:string)  [unwired: 4 in]
      n120 = Concatenate Strings(w419) -> (w418:string)
      n121 = Build Array(w371) -> (w372:string[])
      n122 = Insert Into Array(array=string[][] [] ("text data"), new element=w372) -> (w374:string[][])  [unwired: 2 in]
      n123 = call-poly <vilib>:"Excel Easy Table.vi"("report in"=w369, "start (0, 0)"=cluster{"row":i32, "column":i32} {"row"=22, "column"=20}, "text data"=w374, "error in (no error)"=w368) -> ("report out"=w366:refnum<class "NI_report.lvclass">, "error out"=w367:errorcluster)  [unwired: 7 in, 3 out]
      n124 = call "ExcelReportSubVI.vi"("start (0, 0)"=cluster{"row":i32, "column":i32} {"row"=24, "column"=20}, "error in (no error)"=w367, "Test İn"=w317, "report in"=w366) -> ("error out"=w384:errorcluster, "Table out"=w316:string[][], "report out"=w388:refnum<class "NI_report.lvclass">, "Yazılacak Parametre"=w375:string)  [unwired: 4 in]
      n125 = call "ExcelReportSubVI.vi"("start (0, 0)"=cluster{"row":i32, "column":i32} {"row"=25, "column"=20}, "error in (no error)"=w384, "Test İn"=w316, "report in"=w388) -> ("error out"=w337:errorcluster, "Table out"=w315:string[][], "report out"=w338:refnum<class "NI_report.lvclass">, "Yazılacak Parametre"=w347:string)  [unwired: 4 in]
      n126 = call "ExcelReportSubVI.vi"("start (0, 0)"=cluster{"row":i32, "column":i32} {"row"=27, "column"=20}, "error in (no error)"=w337, "Test İn"=w315, "report in"=w338) -> ("error out"=w339:errorcluster, "Table out"=w314:string[][], "report out"=w340:refnum<class "NI_report.lvclass">, "Yazılacak Parametre"=w334:string)  [unwired: 4 in]
      n127 = call "ExcelReportSubVI.vi"("start (0, 0)"=cluster{"row":i32, "column":i32} {"row"=28, "column"=20}, "error in (no error)"=w339, "Test İn"=w314, "report in"=w340) -> ("error out"=w335:errorcluster, "report out"=w336:refnum<class "NI_report.lvclass">, "Yazılacak Parametre"=w333:string)  [unwired: 4 in, 1 out]
      n128 = Build Array(w363) -> (w362:string[])
      n129 = Insert Into Array(array=string[][] [] ("text data"), new element=w362) -> (w360:string[][])  [unwired: 2 in]
      n130 = call-poly <vilib>:"Excel Easy Table.vi"("report in"=w336, "start (0, 0)"=cluster{"row":i32, "column":i32} {"row"=33, "column"=20}, "text data"=w360, "error in (no error)"=w335) -> ("report out"=w359:refnum<class "NI_report.lvclass">, "error out"=w358:errorcluster)  [unwired: 7 in, 3 out]
      n131 = case shown="True" TRUE {
        tunnel: w418 -> [_ w453]
        tunnel: [w443 w447] -> w417
        tunnel: [w442 w446] -> w416
        tunnel: w359 -> [w443 w445]
        tunnel: w358 -> [w442 w444]
        frame False {
        }
        frame True {
          n132 = Build Array(w453) -> (w454:string[])
          n133 = Insert Into Array(array=string[][] [] ("text data"), new element=w454) -> (w448:string[][])  [unwired: 2 in]
          n134 = Bundle By Name(cluster=T4 {"position (excel)"={"row"=0, "column"=0}, "name (excel)"="", "bookmark (word)"=""} ("MS Office parameters"), "position (excel)"=cluster{"row":i32, "column":i32} {"row"=5, "column"=14} ("start (0, 0)")) -> (w450:T4)
          n135 = call-poly <vilib>:"Append Table to Report.vi"("report in"=w445, "column width (1)"=1.0, "MS Office parameters"=w450, "text data"=w448, "error in (no error)"=w444) -> ("report out"=w447:refnum<class "NI_report.lvclass">, "error out"=w446:errorcluster)  [unwired: 7 in, 2 out]
        }
      }
      n136 = call-dynamic "Save Report to File.vi"("report in"=w417, "report file path"=w343, "prompt to replace? (F)"=FALSE, "error in (no error)"=w416) -> ("error out"=w399:errorcluster)  [unwired: 10 in, 1 out]
      n137 = call <vilib>:"Clear Errors.vi"("error in (no error)"=w399) -> ("error out"=w398:errorcluster)  [unwired: 5 in, 1 out]
    }
    frame 4 {
      # "save"
      n138 = case shown="True" w456 {
        tunnel: [w561 w709] -> w466
        tunnel: w465 -> [w533 w681]
        tunnel: w464 -> [w532 w680]
        tunnel: w463 -> [w531 w679]
        tunnel: [w530 w678] -> w462
        tunnel: _ -> [w529 w677]
        tunnel: _ -> [_ w676]
        tunnel: w461 -> [w519 w666]
        tunnel: w460 -> [w514 w661]
        tunnel: w459 -> [w499 w646]
        tunnel: w458 -> [w476 w621]
        tunnel: [w468 _] -> w457
        frame True {
          w548 = cluster{"row":i32, "column":i32} {"row"=16, "column"=20} ("start (0, 0)")
          w585 = "." ("string")
          # "31"
          # "RPM 11 \nAKIM 12"
          # "sabun"
          n139 = Get Date/Time In Seconds() -> (seconds since 1Jan1904=w592:timestamp)
          n140 = Get Date/Time String(seconds (now)=w592) -> (date string=w582:string, time string=w583:string)  [unwired: 2 in]
          n141 = Select(t="OK" ("worksheet name (\"\")"), s=w531, f="RED" ("worksheet name (\"\")")) -> (s? t:f=w584:string)
          n142 = Search and Replace String(input string=w583, search string=":", replace string="." ("replace string (\"\")")) -> (result string=w578:string)  [unwired: 5 in, 3 out]
          n143 = Number To Fractional String(number=w533, precision (6)=i16 0) -> (F-format string=w568:string)  [unwired: 2 in]
          n144 = call <vilib>:"Create Report.vi"("window state (normal)"=T2."minimized", "report type"=Report_Type."Excel", "template (empty)"=w468, "error in (no error)"=w532) -> ("report out"=w594:refnum<class "NI_report.lvclass">, "error out"=w593:errorcluster)  [unwired: 10 in]
          n145 = Select(t="OK" ("worksheet name (\"\")"), s=w531, f="RED" ("worksheet name (\"\")")) -> (s? t:f=w540:string)
          n146 = Concatenate Strings(w540, "_" ("string"), w514, w585, w582, w585, w578, ".xlsx" ("string")) -> (w589:string)
          n147 = Concatenate Strings(w568, " °C" ("string")) -> (w566:string)
          n148 = call <vilib>:"Excel Rename Worksheet.vi"("report in"=w594, "worksheet name (\"\")"=w584, "error in (no error)"=w593) -> ("report out"=w573:refnum<class "NI_report.lvclass">, "error out"=w572:errorcluster)  [unwired: 11 in]
          n149 = Build Array(w566) -> (w569:string[])
          n150 = Insert Into Array(array=string[][] [] ("text data"), new element=w569) -> (w565:string[][])  [unwired: 2 in]
          n151 = case shown="False" FALSE {
            tunnel: w573 -> [w598 w605]
            tunnel: w572 -> [w597 w604]
            tunnel: cluster{"row":i32, "column":i32} {"row"=4, "column"=14} ("start (0, 0)") -> [_ w603]
            tunnel: w565 -> [_ w602]
            tunnel: [w598 w601] -> w517
            tunnel: [w597 w600] -> w516
            tunnel: [T3 {"font name"="", "font size"=0.0, "bold"=0, "italic"=0, "underline"=0, "strike through"=0, "font color"=16777216} ("font out") w599] -> w515
            frame False {
            }
            frame True {
              n152 = call-poly <vilib>:"Excel Easy Table.vi"("report in"=w605, "start (0, 0)"=w603, "text data"=w602, "error in (no error)"=w604) -> ("report out"=w601:refnum<class "NI_report.lvclass">, "font out"=w599:T3, "error out"=w600:errorcluster)  [unwired: 7 in, 2 out]
            }
          }
          n153 = Build Array(w514) -> (w577:string[])
          n154 = Insert Into Array(array=string[][] [] ("text data"), new element=w577) -> (w576:string[][])  [unwired: 2 in]
          n155 = call-poly <vilib>:"Excel Easy Table.vi"("report in"=w517, "font"=w515, "start (0, 0)"=cluster{"row":i32, "column":i32} {"row"=6, "column"=7}, "text data"=w576, "error in (no error)"=w516) -> ("report out"=w528:refnum<class "NI_report.lvclass">, "error out"=w527:errorcluster)  [unwired: 6 in, 3 out]
          n156 = call "ExcelReportSubVI.vi"("start (0, 0)"=cluster{"row":i32, "column":i32} {"row"=11, "column"=20}, "error in (no error)"=w527, "Test İn"=w519, "report in"=w528) -> ("error out"=w525:errorcluster, "Table out"=w512:string[][], "report out"=w526:refnum<class "NI_report.lvclass">, "Yazılacak Parametre"=w518:string)  [unwired: 4 in]
          n157 = call "ExcelReportSubVI.vi"("start (0, 0)"=cluster{"row":i32, "column":i32} {"row"=12, "column"=20}, "error in (no error)"=w525, "Test İn"=w512, "report in"=w526) -> ("error out"=w523:errorcluster, "Table out"=w511:string[][], "report out"=w524:refnum<class "NI_report.lvclass">, "Yazılacak Parametre"=w520:string)  [unwired: 4 in]
          n158 = Build Path(base path=w529, name or relative path=w589) -> (appended path=w530:path)
          n159 = call "ExcelReportSubVI.vi"("start (0, 0)"=cluster{"row":i32, "column":i32} {"row"=14, "column"=20}, "error in (no error)"=w523, "Test İn"=w511, "report in"=w524) -> ("error out"=w559:errorcluster, "Table out"=w510:string[][], "report out"=w560:refnum<class "NI_report.lvclass">, "Yazılacak Parametre"=w539:string)  [unwired: 4 in]
          n160 = call "ExcelReportSubVI.vi"("start (0, 0)"=cluster{"row":i32, "column":i32} {"row"=15, "column"=20}, "error in (no error)"=w559, "Test İn"=w510, "report in"=w560) -> ("error out"=w557:errorcluster, "Table out"=w509:string[][], "report out"=w558:refnum<class "NI_report.lvclass">, "Yazılacak Parametre"=w538:string)  [unwired: 4 in]
          n161 = call "ExcelReportSubVI.vi"("error in (no error)"=w557, "Test İn"=w509, "report in"=w558) -> ("error out"=w553:errorcluster, "Table out"=w508:string[][], "report out"=w556:refnum<class "NI_report.lvclass">, "start (0, 0)"=w467:cluster{"row":i32, "column":i32}, "Yazılacak Parametre"=w537:string)  [unwired: 4 in]
          n162 = Concatenate Strings(w582) -> (w581:string)
          n163 = call "ExcelReportSubVI.vi"("start (0, 0)"=cluster{"row":i32, "column":i32} {"row"=17, "column"=20}, "error in (no error)"=w553, "Test İn"=w508, "report in"=w556) -> ("error out"=w552:errorcluster, "Table out"=w507:string[][], "report out"=w555:refnum<class "NI_report.lvclass">, "Yazılacak Parametre"=w536:string)  [unwired: 4 in]
          n164 = call "ExcelReportSubVI.vi"("start (0, 0)"=cluster{"row":i32, "column":i32} {"row"=18, "column"=20}, "error in (no error)"=w552, "Test İn"=w507, "report in"=w555) -> ("error out"=w551:errorcluster, "Table out"=w506:string[][], "report out"=w554:refnum<class "NI_report.lvclass">, "Yazılacak Parametre"=w535:string)  [unwired: 4 in]
          n165 = call "ExcelReportSubVI.vi"("start (0, 0)"=cluster{"row":i32, "column":i32} {"row"=19, "column"=20}, "error in (no error)"=w551, "Test İn"=w506, "report in"=w554) -> ("error out"=w495:errorcluster, "Table out"=w505:string[][], "report out"=w497:refnum<class "NI_report.lvclass">, "Yazılacak Parametre"=w534:string)  [unwired: 4 in]
          n166 = call "ExcelReportSubVI.vi"("start (0, 0)"=cluster{"row":i32, "column":i32} {"row"=21, "column"=20}, "error in (no error)"=w495, "Test İn"=w505, "report in"=w497) -> ("error out"=w494:errorcluster, "Table out"=w487:string[][], "report out"=w496:refnum<class "NI_report.lvclass">, "Yazılacak Parametre"=w503:string)  [unwired: 4 in]
          n167 = Build Array(w499) -> (w498:string[])
          n168 = Insert Into Array(array=string[][] [] ("text data"), new element=w498) -> (w501:string[][])  [unwired: 2 in]
          n169 = call-poly <vilib>:"Excel Easy Table.vi"("report in"=w496, "start (0, 0)"=cluster{"row":i32, "column":i32} {"row"=23, "column"=20}, "text data"=w501, "error in (no error)"=w494) -> ("report out"=w486:refnum<class "NI_report.lvclass">, "error out"=w485:errorcluster)  [unwired: 7 in, 3 out]
          n170 = call "ExcelReportSubVI.vi"("start (0, 0)"=cluster{"row":i32, "column":i32} {"row"=25, "column"=20}, "error in (no error)"=w485, "Test İn"=w487, "report in"=w486) -> ("error out"=w491:errorcluster, "Table out"=w490:string[][], "report out"=w492:refnum<class "NI_report.lvclass">, "Yazılacak Parametre"=w488:string)  [unwired: 4 in]
          n171 = call "ExcelReportSubVI.vi"("start (0, 0)"=cluster{"row":i32, "column":i32} {"row"=26, "column"=20}, "error in (no error)"=w491, "Test İn"=w490, "report in"=w492) -> ("error out"=w477:errorcluster, "Table out"=w469:string[][], "report out"=w478:refnum<class "NI_report.lvclass">, "Yazılacak Parametre"=w489:string)  [unwired: 4 in]
          n172 = Build Array(w476) -> (w482:string[])
          n173 = Insert Into Array(array=string[][] [] ("text data"), new element=w482) -> (w481:string[][])  [unwired: 2 in]
          n174 = call-poly <vilib>:"Excel Easy Table.vi"("report in"=w478, "start (0, 0)"=cluster{"row":i32, "column":i32} {"row"=31, "column"=20}, "text data"=w481, "error in (no error)"=w477) -> ("report out"=w473:refnum<class "NI_report.lvclass">, "error out"=w472:errorcluster)  [unwired: 7 in, 3 out]
          n175 = call "ExcelReportSubVI.vi"("start (0, 0)"=cluster{"row":i32, "column":i32} {"row"=34, "column"=20}, "error in (no error)"=w472, "Test İn"=w469, "report in"=w473) -> ("error out"=w471:errorcluster, "report out"=w470:refnum<class "NI_report.lvclass">, "Yazılacak Parametre"=w474:string)  [unwired: 4 in, 1 out]
          n176 = case shown="True" TRUE {
            tunnel: w581 -> [_ w617]
            tunnel: [w607 w611] -> w580
            tunnel: [w606 w610] -> w579
            tunnel: w470 -> [w607 w609]
            tunnel: w471 -> [w606 w608]
            frame False {
            }
            frame True {
              n177 = Build Array(w617) -> (w618:string[])
              n178 = Insert Into Array(array=string[][] [] ("text data"), new element=w618) -> (w612:string[][])  [unwired: 2 in]
              n179 = Bundle By Name(cluster=T4 {"position (excel)"={"row"=0, "column"=0}, "name (excel)"="", "bookmark (word)"=""} ("MS Office parameters"), "position (excel)"=cluster{"row":i32, "column":i32} {"row"=5, "column"=14} ("start (0, 0)")) -> (w614:T4)
              n180 = call-poly <vilib>:"Append Table to Report.vi"("report in"=w609, "column width (1)"=1.0, "MS Office parameters"=w614, "text data"=w612, "error in (no error)"=w608) -> ("report out"=w611:refnum<class "NI_report.lvclass">, "error out"=w610:errorcluster)  [unwired: 7 in, 2 out]
            }
          }
          n181 = call-dynamic "Save Report to File.vi"("report in"=w580, "report file path"=w530, "prompt to replace? (F)"=FALSE, "error in (no error)"=w579) -> ("error out"=w562:errorcluster)  [unwired: 10 in, 1 out]
          n182 = call <vilib>:"Clear Errors.vi"("error in (no error)"=w562) -> ("error out"=w561:errorcluster)  [unwired: 5 in, 1 out]
        }
        frame False {
          w696 = cluster{"row":i32, "column":i32} {"row"=16, "column"=20} ("start (0, 0)")
          w733 = "." ("string")
          # "31"
          # "RPM 11 \nAKIM 12"
          # "sabun"
          n183 = Get Date/Time In Seconds() -> (seconds since 1Jan1904=w740:timestamp)
          n184 = Get Date/Time String(seconds (now)=w740) -> (date string=w730:string, time string=w731:string)  [unwired: 2 in]
          n185 = Select(t="OK" ("worksheet name (\"\")"), s=w679, f="RED" ("worksheet name (\"\")")) -> (s? t:f=w732:string)
          n186 = Search and Replace String(input string=w731, search string=":", replace string="." ("replace string (\"\")")) -> (result string=w726:string)  [unwired: 5 in, 3 out]
          n187 = Number To Fractional String(number=w681, precision (6)=i16 0) -> (F-format string=w716:string)  [unwired: 2 in]
          n188 = call <vilib>:"Create Report.vi"("window state (normal)"=T2."minimized", "report type"=Report_Type."Excel", "template (empty)"=w676, "error in (no error)"=w680) -> ("report out"=w742:refnum<class "NI_report.lvclass">, "error out"=w741:errorcluster)  [unwired: 10 in]
          n189 = Select(t="OK" ("worksheet name (\"\")"), s=w679, f="RED" ("worksheet name (\"\")")) -> (s? t:f=w688:string)
          n190 = Concatenate Strings(w688, "_" ("string"), w661, w733, w730, w733, w726, ".xlsx" ("string")) -> (w737:string)
          n191 = Concatenate Strings(w716, " °C" ("string")) -> (w714:string)
          n192 = call <vilib>:"Excel Rename Worksheet.vi"("report in"=w742, "worksheet name (\"\")"=w732, "error in (no error)"=w741) -> ("report out"=w721:refnum<class "NI_report.lvclass">, "error out"=w720:errorcluster)  [unwired: 11 in]
          n193 = Build Array(w714) -> (w717:string[])
          n194 = Insert Into Array(array=string[][] [] ("text data"), new element=w717) -> (w713:string[][])  [unwired: 2 in]
          n195 = case shown="False" FALSE {
            tunnel: w721 -> [w746 w753]
            tunnel: w720 -> [w745 w752]
            tunnel: cluster{"row":i32, "column":i32} {"row"=4, "column"=14} ("start (0, 0)") -> [_ w751]
            tunnel: w713 -> [_ w750]
            tunnel: [w746 w749] -> w664
            tunnel: [w745 w748] -> w663
            tunnel: [T3 {"font name"="", "font size"=0.0, "bold"=0, "italic"=0, "underline"=0, "strike through"=0, "font color"=16777216} ("font out") w747] -> w662
            frame False {
            }
            frame True {
              n196 = call-poly <vilib>:"Excel Easy Table.vi"("report in"=w753, "start (0, 0)"=w751, "text data"=w750, "error in (no error)"=w752) -> ("report out"=w749:refnum<class "NI_report.lvclass">, "font out"=w747:T3, "error out"=w748:errorcluster)  [unwired: 7 in, 2 out]
            }
          }
          n197 = Build Array(w661) -> (w725:string[])
          n198 = Insert Into Array(array=string[][] [] ("text data"), new element=w725) -> (w724:string[][])  [unwired: 2 in]
          n199 = call-poly <vilib>:"Excel Easy Table.vi"("report in"=w664, "font"=w662, "start (0, 0)"=cluster{"row":i32, "column":i32} {"row"=6, "column"=7}, "text data"=w724, "error in (no error)"=w663) -> ("report out"=w675:refnum<class "NI_report.lvclass">, "error out"=w674:errorcluster)  [unwired: 6 in, 3 out]
          n200 = call "ExcelReportSubVI.vi"("start (0, 0)"=cluster{"row":i32, "column":i32} {"row"=11, "column"=20}, "error in (no error)"=w674, "Test İn"=w666, "report in"=w675) -> ("error out"=w672:errorcluster, "Table out"=w659:string[][], "report out"=w673:refnum<class "NI_report.lvclass">, "Yazılacak Parametre"=w665:string)  [unwired: 4 in]
          n201 = call "ExcelReportSubVI.vi"("start (0, 0)"=cluster{"row":i32, "column":i32} {"row"=12, "column"=20}, "error in (no error)"=w672, "Test İn"=w659, "report in"=w673) -> ("error out"=w670:errorcluster, "Table out"=w658:string[][], "report out"=w671:refnum<class "NI_report.lvclass">, "Yazılacak Parametre"=w667:string)  [unwired: 4 in]
          n202 = Build Path(base path=w677, name or relative path=w737) -> (appended path=w678:path)
          n203 = call "ExcelReportSubVI.vi"("start (0, 0)"=cluster{"row":i32, "column":i32} {"row"=14, "column"=20}, "error in (no error)"=w670, "Test İn"=w658, "report in"=w671) -> ("error out"=w707:errorcluster, "Table out"=w657:string[][], "report out"=w708:refnum<class "NI_report.lvclass">, "Yazılacak Parametre"=w687:string)  [unwired: 4 in]
          n204 = call "ExcelReportSubVI.vi"("start (0, 0)"=cluster{"row":i32, "column":i32} {"row"=15, "column"=20}, "error in (no error)"=w707, "Test İn"=w657, "report in"=w708) -> ("error out"=w705:errorcluster, "Table out"=w656:string[][], "report out"=w706:refnum<class "NI_report.lvclass">, "Yazılacak Parametre"=w686:string)  [unwired: 4 in]
          n205 = call "ExcelReportSubVI.vi"("error in (no error)"=w705, "Test İn"=w656, "report in"=w706) -> ("error out"=w701:errorcluster, "Table out"=w655:string[][], "report out"=w704:refnum<class "NI_report.lvclass">, "start (0, 0)"=w620:cluster{"row":i32, "column":i32}, "Yazılacak Parametre"=w685:string)  [unwired: 4 in]
          n206 = Concatenate Strings(w730) -> (w729:string)
          n207 = call "ExcelReportSubVI.vi"("start (0, 0)"=cluster{"row":i32, "column":i32} {"row"=17, "column"=20}, "error in (no error)"=w701, "Test İn"=w655, "report in"=w704) -> ("error out"=w700:errorcluster, "Table out"=w654:string[][], "report out"=w703:refnum<class "NI_report.lvclass">, "Yazılacak Parametre"=w684:string)  [unwired: 4 in]
          n208 = call "ExcelReportSubVI.vi"("start (0, 0)"=cluster{"row":i32, "column":i32} {"row"=18, "column"=20}, "error in (no error)"=w700, "Test İn"=w654, "report in"=w703) -> ("error out"=w699:errorcluster, "Table out"=w653:string[][], "report out"=w702:refnum<class "NI_report.lvclass">, "Yazılacak Parametre"=w683:string)  [unwired: 4 in]
          n209 = call "ExcelReportSubVI.vi"("start (0, 0)"=cluster{"row":i32, "column":i32} {"row"=19, "column"=20}, "error in (no error)"=w699, "Test İn"=w653, "report in"=w702) -> ("error out"=w642:errorcluster, "Table out"=w652:string[][], "report out"=w644:refnum<class "NI_report.lvclass">, "Yazılacak Parametre"=w682:string)  [unwired: 4 in]
          n210 = call "ExcelReportSubVI.vi"("start (0, 0)"=cluster{"row":i32, "column":i32} {"row"=21, "column"=20}, "error in (no error)"=w642, "Test İn"=w652, "report in"=w644) -> ("error out"=w641:errorcluster, "Table out"=w634:string[][], "report out"=w643:refnum<class "NI_report.lvclass">, "Yazılacak Parametre"=w650:string)  [unwired: 4 in]
          n211 = Build Array(w646) -> (w645:string[])
          n212 = Insert Into Array(array=string[][] [] ("text data"), new element=w645) -> (w648:string[][])  [unwired: 2 in]
          n213 = call-poly <vilib>:"Excel Easy Table.vi"("report in"=w643, "start (0, 0)"=cluster{"row":i32, "column":i32} {"row"=23, "column"=20}, "text data"=w648, "error in (no error)"=w641) -> ("report out"=w633:refnum<class "NI_report.lvclass">, "error out"=w632:errorcluster)  [unwired: 7 in, 3 out]
          n214 = call "ExcelReportSubVI.vi"("start (0, 0)"=cluster{"row":i32, "column":i32} {"row"=25, "column"=20}, "error in (no error)"=w632, "Test İn"=w634, "report in"=w633) -> ("error out"=w638:errorcluster, "Table out"=w637:string[][], "report out"=w639:refnum<class "NI_report.lvclass">, "Yazılacak Parametre"=w635:string)  [unwired: 4 in]
          n215 = call "ExcelReportSubVI.vi"("start (0, 0)"=cluster{"row":i32, "column":i32} {"row"=26, "column"=20}, "error in (no error)"=w638, "Test İn"=w637, "report in"=w639) -> ("error out"=w624:errorcluster, "report out"=w625:refnum<class "NI_report.lvclass">, "Yazılacak Parametre"=w636:string)  [unwired: 4 in, 1 out]
          n216 = Build Array(w621) -> (w629:string[])
          n217 = Insert Into Array(array=string[][] [] ("text data"), new element=w629) -> (w628:string[][])  [unwired: 2 in]
          n218 = call-poly <vilib>:"Excel Easy Table.vi"("report in"=w625, "start (0, 0)"=cluster{"row":i32, "column":i32} {"row"=31, "column"=20}, "text data"=w628, "error in (no error)"=w624) -> ("report out"=w623:refnum<class "NI_report.lvclass">, "error out"=w622:errorcluster)  [unwired: 7 in, 3 out]
          n219 = case shown="True" TRUE {
            tunnel: w729 -> [_ w765]
            tunnel: [w755 w759] -> w728
            tunnel: [w754 w758] -> w727
            tunnel: w623 -> [w755 w757]
            tunnel: w622 -> [w754 w756]
            frame False {
            }
            frame True {
              n220 = Build Array(w765) -> (w766:string[])
              n221 = Insert Into Array(array=string[][] [] ("text data"), new element=w766) -> (w760:string[][])  [unwired: 2 in]
              n222 = Bundle By Name(cluster=T4 {"position (excel)"={"row"=0, "column"=0}, "name (excel)"="", "bookmark (word)"=""} ("MS Office parameters"), "position (excel)"=cluster{"row":i32, "column":i32} {"row"=5, "column"=14} ("start (0, 0)")) -> (w762:T4)
              n223 = call-poly <vilib>:"Append Table to Report.vi"("report in"=w757, "column width (1)"=1.0, "MS Office parameters"=w762, "text data"=w760, "error in (no error)"=w756) -> ("report out"=w759:refnum<class "NI_report.lvclass">, "error out"=w758:errorcluster)  [unwired: 7 in, 2 out]
            }
          }
          n224 = call-dynamic "Save Report to File.vi"("report in"=w728, "report file path"=w678, "prompt to replace? (F)"=FALSE, "error in (no error)"=w727) -> ("error out"=w710:errorcluster)  [unwired: 10 in, 1 out]
          n225 = call <vilib>:"Clear Errors.vi"("error in (no error)"=w710) -> ("error out"=w709:errorcluster)  [unwired: 5 in, 1 out]
        }
      }
    }
  }
  "error out" <- w17
  "appended path" <- w5
